vi "GetOldData.vi"(11 "LogPath":path) -> (1 "log":string, 2 "clients":string, 3 "server":string)   [LabVIEW 2012]
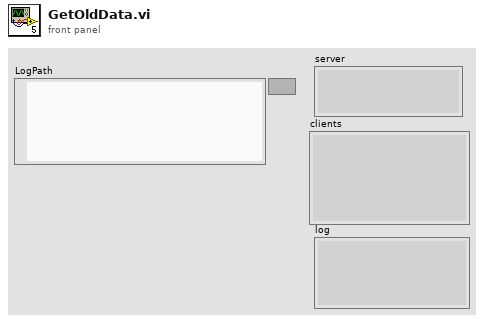
[diagram p1: front panel]
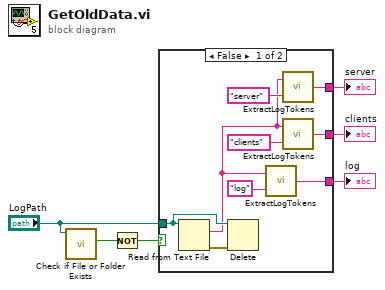
[diagram p0: block diagram]
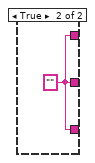
[diagram p2: hidden frame]
diagram:
  n1 = call <vilib>:"Check if File or Folder Exists.vi"("path"="LogPath") -> ("file or folder exists?"=w2:bool)  [unwired: 8 in, 2 out]
  n2 = Not(x=w2) -> (.not. x?=w3:bool)
  n3 = case shown="False" w3 {
    tunnel: "LogPath" -> [w14 _]
    tunnel: [w12 w16] -> w6
    tunnel: [w10 w16] -> w1
    tunnel: [w7 w16] -> w5
    frame False {
      n4 = Read from Text File(file (use dialog)=w14) -> (text=w8:string, error out=w15:errorcluster)  [unwired: 3 in, 2 out]
      n5 = Delete(path (use dialog)=w14, error in=w15) -> ()  [unwired: 3 in, 3 out]
      n6 = call <userlib>:"ExtractLogTokens.vi"("HTML"=w8, "section"="log" ("string")) -> ("tagged text"=w12:string)  [unwired: 2 out]
      n7 = call <userlib>:"ExtractLogTokens.vi"("HTML"=w8, "section"="server" ("string")) -> ("tagged text"=w10:string)  [unwired: 2 out]
      n8 = call <userlib>:"ExtractLogTokens.vi"("HTML"=w8, "section"="clients" ("string")) -> ("tagged text"=w7:string)  [unwired: 2 out]
    }
    frame True {
      w16 = ""
    }
  }
  "log" <- w6
  "clients" <- w5
  "server" <- w1
